vi "Test Arm.vi"() -> ()   [LabVIEW 2015]
panel:
  out "Array":dbl[](array[numeric])
  in  "Rate Control K 2":dbl
  in  "Desired Coordinates 2":cluster{"x":dbl, "y":dbl}
  out "appended array":dbl[](array[numeric])
  out "Desired angle at 1":dbl(graph)
  out "Desired angle at S":dbl(graph)
  out "Current X":dbl
  out "Current Y":dbl
  in  "Encoders":cluster{"encoder at S":dbl, "encoder at 1":dbl}
  out "Desired angle at Shoulder":dbl
  out "Desired angle at 1":dbl
  out "Distance from Base to setpoint":dbl
  out "angle at 1":dbl
  out "angle at S":dbl
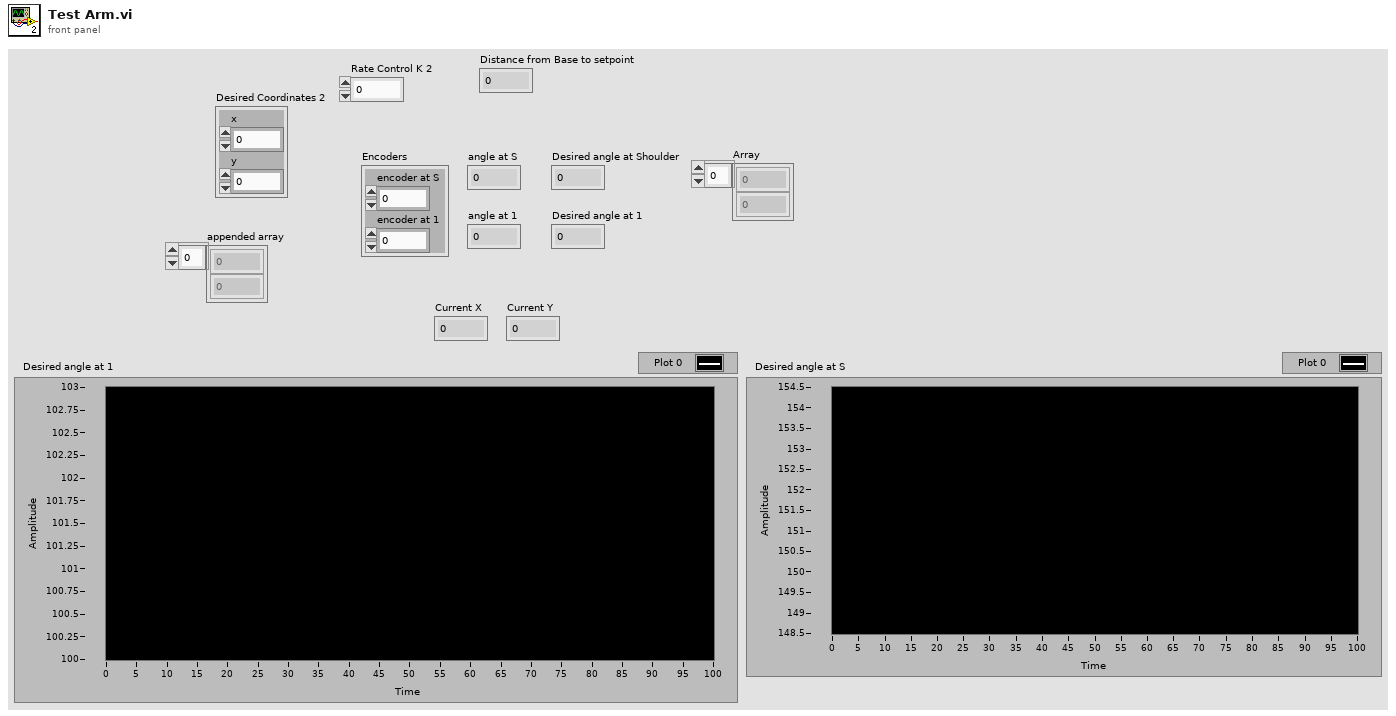
[diagram p1: front panel]
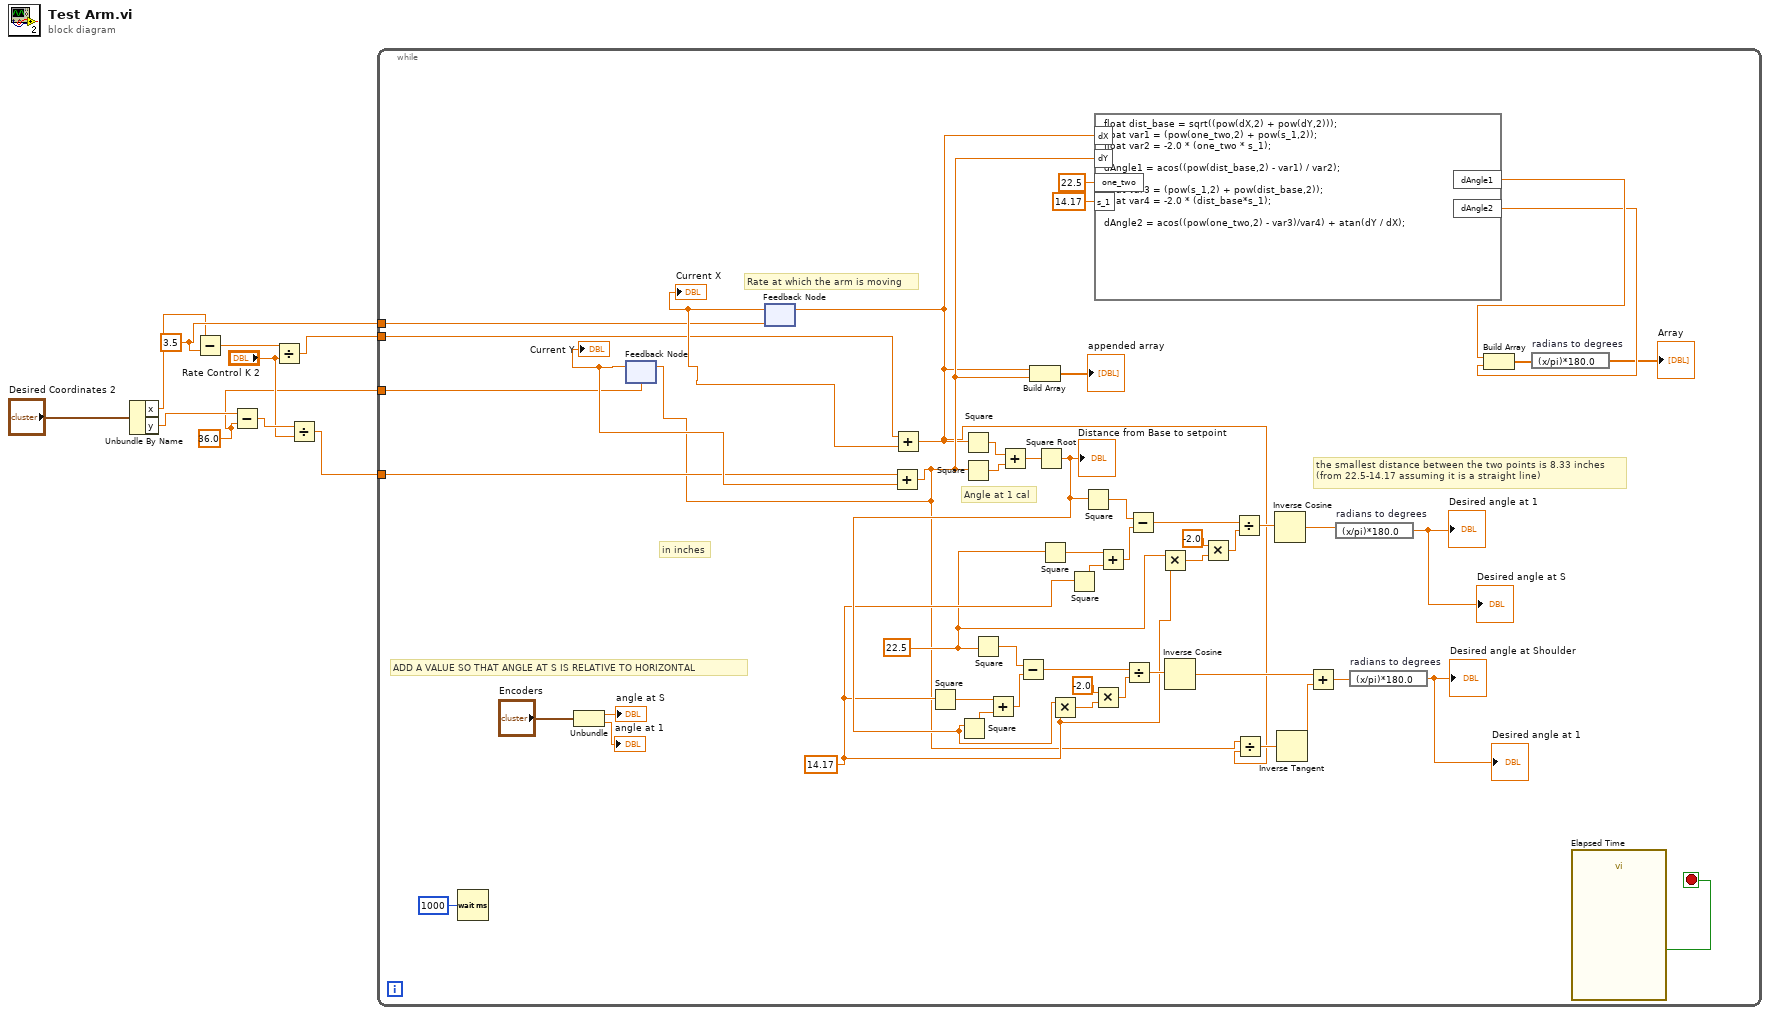
[diagram p0: block diagram]
diagram:
  w1 = 36.0 ("x")
  w3 = 3.5 ("x")
  n1 = Unbundle By Name("Desired Coordinates 2") -> ("x"=w2:dbl, "y"=w4:dbl)
  n2 = Subtract(x=w2, y=w3) -> (x-y=w9:dbl)
  n3 = Subtract(x=w4, y=w1) -> (x-y=w8:dbl)
  n4 = Divide(x=w9, y="Rate Control K 2") -> (x/y=w6:dbl)
  n5 = Divide(x=w8, y="Rate Control K 2") -> (x/y=w5:dbl)
  n6 = while {
    tunnel: w6 -> [w26]
    tunnel: w5 -> [w25]
    tunnel: w3 -> [w24]
    tunnel: w1 -> [w23]
    stop <- w22 stop-if-true
    w19 = 22.5 ("x")
    w20 = 14.17 ("S - 1")
    # "Rate at which the arm is moving"
    # "ADD A VALUE SO THAT ANGLE AT S IS RELATIVE TO HORIZONTAL"
    # "the smallest distance between the two points is 8.33 inches\n(from 22.5-14.17 assuming it is a straight line)"
    # "Angle at 1 cal"
    # "in inches"
    n7 = Wait (ms)(milliseconds to wait=u32 1000) -> ()  [unwired: 1 out]
    n8 = Unbundle("Encoders") -> ("encoder at S"=→"angle at S":dbl, "encoder at 1"=→"angle at 1":dbl)
    n9 = feedback #1(w23) -> (w32:dbl)
    "Current Y" <- w32
    n10 = feedback #2(w24) -> (w31:dbl)
    "Current X" <- w31
    n11 = Add(x=w25, y=w32) -> (x+y=w16:dbl)
    n12 = feedback-in #1(w16) -> ()
    n13 = Add(x=w26, y=w31) -> (x+y=w15:dbl)
    n14 = feedback-in #2(w15) -> ()
    n15 = Square(x=w20) -> (x^2=w43:dbl)
    n16 = Square(x=w15) -> (x^2=w61:dbl)
    n17 = Square(x=w16) -> (x^2=w60:dbl)
    n18 = Square(x=w19) -> (x^2=w41:dbl)
    n19 = Add(x=w61, y=w60) -> (x+y=w59:dbl)
    n20 = Build Array(w15, w16) -> (→"appended array":dbl[])
    n21 = Square Root(x=w59) -> (sqrt(x)=w21:dbl)
    "Distance from Base to setpoint" <- w21
    n22 = Square(x=w21) -> (x^2=w42:dbl)
    n23 = Add(x=w43, y=w42) -> (x+y=w44:dbl)
    n24 = Subtract(x=w41, y=w44) -> (x-y=w47:dbl)
    n25 = Square(x=w19) -> (x^2=w56:dbl)
    n26 = Multiply(x=w21, y=w20) -> (x*y=w46:dbl)
    n27 = Square(x=w20) -> (x^2=w57:dbl)
    n28 = Square(x=w21) -> (x^2=w58:dbl)
    n29 = Multiply(x=-2.0, y=w46) -> (x*y=w48:dbl)
    n30 = formula code="float dist_base = sqrt((pow(dX,2) + pow(dY,2)));\nfloat var1 = (pow(one_two,2) + pow(s_1,2));\nfloat var2 = -2.0 * (one_two * s_1);\n\ndAngle1 = acos((pow(dist_base,2) - var1) / var2);\n\nfloat var3 = (pow(s_1,2) + pow(dist_base,2));\nfloat var4 = -2.0 * (dist_base*s_1);\n\ndAngle2 = acos((pow(one_two,2) - var3)/var4) + atan(dY / dX);"("dX"=w15, "dY"=w16, "one_two"=22.5 ("input variable"), "s_1"=14.17 ("input variable")) -> ("dAngle1"=w14:dbl, "dAngle2"=w13:dbl)
    n31 = Add(x=w56, y=w57) -> (x+y=w55:dbl)
    n32 = Divide(x=w47, y=w48) -> (x/y=w49:dbl)
    n33 = Subtract(x=w58, y=w55) -> (x-y=w52:dbl)
    n34 = Multiply(x=w19, y=w20) -> (x*y=w53:dbl)
    n35 = Inverse Cosine(1:w49) -> (0:w39:dbl)
    n36 = Multiply(x=-2.0, y=w53) -> (x*y=w51:dbl)
    n37 = Divide(x=w52, y=w51) -> (x/y=w50:dbl)
    n38 = Divide(x=w16, y=w15) -> (x/y=w40:dbl)
    n39 = Inverse Cosine(1:w50) -> (0:w37:dbl)
    n40 = Inverse Tangent(1:w40) -> (0:w38:dbl)
    n41 = Add(x=w39, y=w38) -> (x+y=w36:dbl)
    n42 = expression code="(x/pi)*180.0" "radians to degrees"(w37) -> (→"Desired angle at 1" →"Desired angle at S":dbl)
    n43 = expression code="(x/pi)*180.0" "radians to degrees"(w36) -> (→"Desired angle at Shoulder" →"Desired angle at 1":dbl)
    n44 = Build Array(w14, w13) -> (w12:dbl[])
    n45 = expression code="(x/pi)*180.0" "radians to degrees"(w12) -> (→"Array":dbl[])
    n46 = call "Elapsed Time"() -> ("Time has Elapsed"=w22:bool)  [unwired: 12 in, 7 out]
  }
